vi "Add.vi"(9 "b":dbl=5.0 format="%#_13g", 10 "a":dbl=5.0 format="%#_13g", 11 "LabVIEW Web Service Request":refnum<class "Web Request.lvclass">) -> ()   [LabVIEW 2019]
uses:
  <vilib>/wsapi/Web Request.lvclass
panel:
  out "JSON string":string
  # "Use the Web Service Request input terminal to call the VIs on the Web Services palette. Do not remove it from the connector pane unless you don't need access to the palette."
  # "Each additional control wired to the connector pane will be available as an input in the URL. To include an indicator in terminal-mode output (the default setting), it must also be wired to the connector pane."
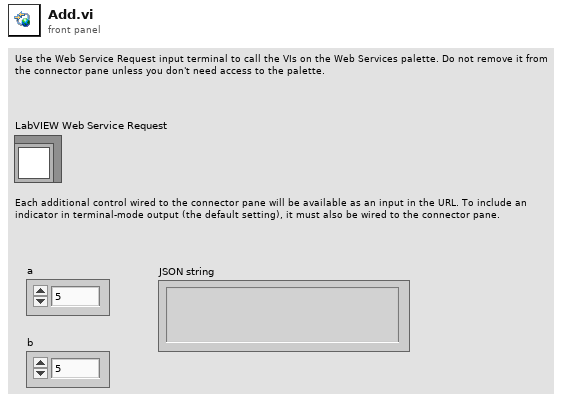
[diagram p1: front panel]
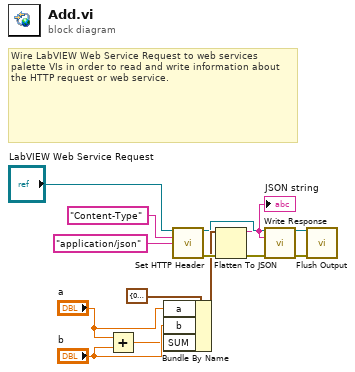
[diagram p0: block diagram]
diagram:
  # "Wire LabVIEW Web Service Request to web services palette VIs in order to read and write information about the HTTP request or web service."
  n1 = Add(x="a", y="b") -> (x+y=w6:dbl)
  n2 = Bundle By Name(cluster=cluster{"a":dbl, "b":dbl, "SUM":dbl} {"a"=0.0, "b"=0.0, "SUM"=0.0} ("Cluster"), "a"="a", "b"="b", "SUM"=w6) -> (w7:cluster{"a":dbl, "b":dbl, "SUM":dbl})
  n3 = call <vilib>:"Set HTTP Header.vi"("LabVIEW Web Service Request"="LabVIEW Web Service Request", "header"="Content-Type", "header value"="application/json") -> ("LabVIEW Web Service Request out"=w5:refnum<class "Web Request.lvclass">, "error out"=w12:errorcluster)  [unwired: 11 in]
  n4 = Flatten To JSON(anything=w7, error in (no error)=w12) -> (JSON string=w4:string, 11:w3:errorcluster)  [unwired: 1 in]
  "JSON string" <- w4
  n5 = call <vilib>:"Write Response.vi"("LabVIEW Web Service Request"=w5, "response string"=w4, "error in (no error)"=w3) -> ("LabVIEW Web Service Request out"=w2:refnum<class "Web Request.lvclass">, "error out"=w1:errorcluster)  [unwired: 11 in]
  n6 = call <vilib>:"Flush Output.vi"("LabVIEW Web Service Request"=w2, "error in (no error)"=w1) -> ()  [unwired: 12 in, 2 out]
